vi "VAI Read Datas.vi"(7 "pData":u16, 9 "DataNum":u16, 10 "DevIndex":i32, 11 "DevType":i32) -> (3 "function return":i32, 5 "pData out":u16)   [LabVIEW 2010, in "ControlADC.lvlib"]
doc: "int WINAPI VAI_ReadDatas(int DevType,int DevIndex,unsigned short DataNum,unsigned short *pData);"
uses:
  ControlADC.lvlib
  ControlADC/Ginkgo_Driver.dll
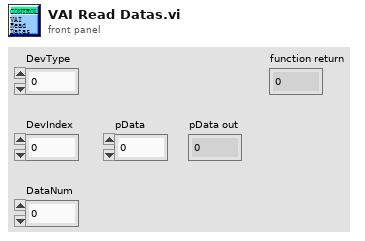
[diagram p1: front panel]
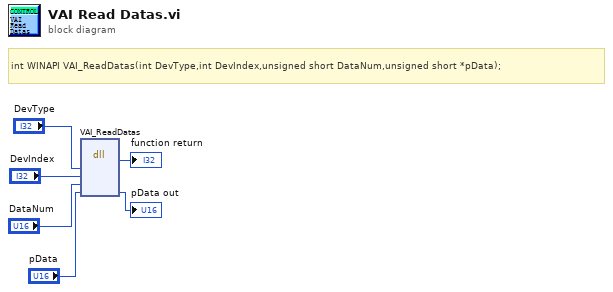
[diagram p0: block diagram]
diagram:
  # "int WINAPI VAI_ReadDatas(int DevType,int DevIndex,unsigned short DataNum,unsigned short *pData);"
  n1 = dll-call lib="E:/Project/vt_ginkgo/truck/Ginkgo Driver/vs2010/Ginkgo_USB-I2C&SPI&CAN_API_v2.0.3.3/lib/labview_32bit/ControlADC/Ginkgo_Driver.*" fn="VAI_ReadDatas"("DevType"="DevType", "DevIndex"="DevIndex", "DataNum"="DataNum", "pData"="pData") -> (→"function return":i32, "pData"=→"pData out":u16)  [unwired: 6 in, 2 out]
